vi "som_deel2 (SubVI).vi"(11 "array":dbl[](array[numeric])) -> (3 "x+y":dbl)   [LabVIEW 2019]
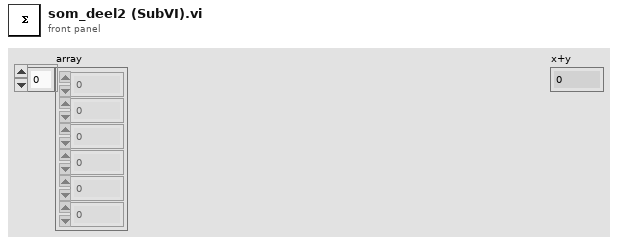
[diagram p1: front panel]
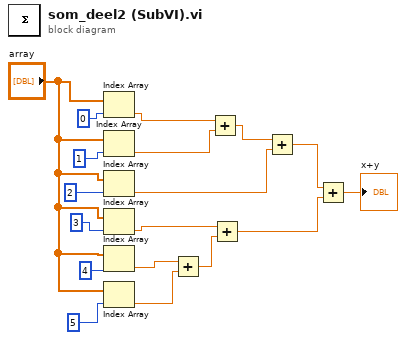
[diagram p0: block diagram]
diagram:
  n1 = Index Array(array="array", index=0) -> (element=w7:dbl)
  n2 = Index Array(array="array", index=1) -> (element=w6:dbl)
  n3 = Index Array(array="array", index=2) -> (element=w4:dbl)
  n4 = Index Array(array="array", index=3) -> (element=w9:dbl)
  n5 = Index Array(array="array", index=4) -> (element=w10:dbl)
  n6 = Index Array(array="array", index=5) -> (element=w11:dbl)
  n7 = Add(x=w10, y=w11) -> (x+y=w8:dbl)
  n8 = Add(x=w7, y=w6) -> (x+y=w5:dbl)
  n9 = Add(x=w9, y=w8) -> (x+y=w2:dbl)
  n10 = Add(x=w5, y=w4) -> (x+y=w3:dbl)
  n11 = Add(x=w3, y=w2) -> (x+y=→"x+y":dbl)
